vi "Read and Send Configuration.vi"(8 "error in (no error)":errorcluster, 9 "Intrs":T2, 10 "Excitation":T1, 11 "MSS Host Actor in":refnum<class "MSS Host Actor.lvclass">) -> (0 "error out":errorcluster, 3 "MSS Host Actor out":refnum<class "MSS Host Actor.lvclass">)   [LabVIEW 2023, in "MSS Host Actor.lvlib" / "MSS Host Actor.lvclass"]
uses:
  MSS Host Actor.lvclass
  ILock-In Remote Actor/ILock-In Remote Actor Messages/Init Msg/Init Msg.lvclass/Init Msg.ctl
  <vilib>/ActorFramework/Message Enqueuer/Message Enqueuer.lvclass/Message Enqueuer.ctl
  <vilib>/ActorFramework/Message Enqueuer/Enqueue.vi
  ILock-In Remote Actor/ILock-In Remote Actor Messages/Init Msg/Init Msg.lvclass
  <vilib>/Utility/error.llb/Error Cluster From Error Code.vi
  <vilib>/ActorFramework/Message Priority Queue/Priority Enqueue.vi
  <vilib>/ErrorRing/Error Ring.xnode
  <vilib>/JDP Science/JSONtext/Config Files/Config File.lvclass
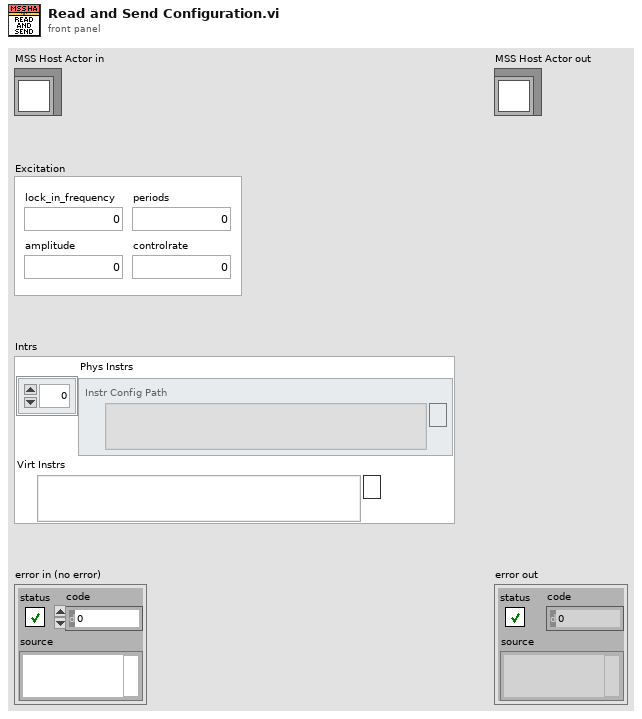
[diagram p1: front panel]
types:
  T1 = cluster{"lock_in_frequency":dbl, "amplitude":dbl, "periods":dbl, "controlrate":dbl}
  T2 = cluster{"Phys Instrs":path[], "Virt Instrs":path}
  T3 = cluster{"Phys Instr CFGs":string[], "Virt Instrs CFG":string}
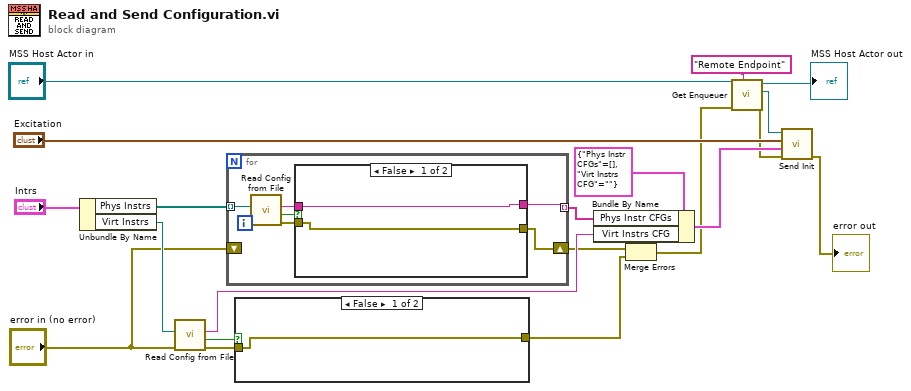
[diagram p0: block diagram]
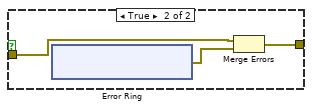
[diagram p2: hidden frame]
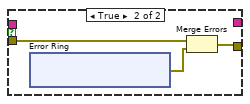
[diagram p3: hidden frame]
diagram:
  n1 = Unbundle By Name("Intrs") -> ("Phys Instrs"=w19:path[], "Virt Instrs"=w18:path)
  n2 = call <vilib>:"Read Config from File.vi"("error in (no error)"="error in (no error)", "config file path"=w18) -> ("error out"=w10:errorcluster, "Template Used (file missing or corrupted)"=w12:bool, "<JSON>Config"=w17:string)  [unwired: 6 in, 1 out]
  n3 = for {
    tunnel: w19 -> [w26] mode=indexing
    shift-right: [w23] -> w13
    shift-left: "error in (no error)" -> [_]
    tunnel: [w22] -> w9 mode=indexing
    n4 = call <vilib>:"Read Config from File.vi"("config file path"=w26) -> ("error out"=w24:errorcluster, "Template Used (file missing or corrupted)"=w25:bool, "<JSON>Config"=w21:string)  [unwired: 7 in, 1 out]
    n5 = case shown="False" w25 {
      tunnel: w24 -> [w27 w30]
      tunnel: w21 -> [w28 _]
      tunnel: [w28 _] -> w22
      tunnel: [w27 w29] -> w23
      frame False {
      }
      frame True {
        n6 = xnode "Error Ring"() -> ("error out"=w31:errorcluster)
        n7 = Merge Errors(w30, w31) -> (w29:errorcluster)
      }
    }
  }
  n8 = case shown="False" w12 {
    tunnel: w10 -> [w37 w39]
    tunnel: [w37 w38] -> w8
    frame False {
    }
    frame True {
      n9 = xnode "Error Ring"() -> ("error out"=w40:errorcluster)
      n10 = Merge Errors(w39, w40) -> (w38:errorcluster)
    }
  }
  n11 = Bundle By Name(cluster=T3 {"Phys Instr CFGs"=[], "Virt Instrs CFG"=""} ("Intrs Configs"), "Phys Instr CFGs"=w9, "Virt Instrs CFG"=w17) -> (w14:T3)
  n12 = Merge Errors(w13, w8) -> (w3:errorcluster)
  n13 = call-dynamic "Get Enqueuer.vi"("Enqueuer Ident"="Remote Endpoint", "error in (no error)"=w3, "My Actor in"="MSS Host Actor in") -> ("error out"=w2:errorcluster, "Nested Actor's Enqueuer"=w4:refnum<class "Message Enqueuer.lvclass">, "My Actor out"=→"MSS Host Actor out":refnum<class "MSS Host Actor.lvclass">)  [unwired: 6 in]
  n14 = call "Send Init.vi"("error in (no error)"=w2, "Intrs Configs"=w14, "Excitation"="Excitation", "Message Enqueuer"=w4) -> ("error out"=→"error out":errorcluster)  [unwired: 6 in, 1 out]
